vi "WF phase diversity_MATLAB_Correction_loop_1_Multi_3.vi"() -> ()   [LabVIEW 2018]
uses:
  Casao LabVIEW SDK 1.0.5/Casao/Casao/Casao.ctl
  <vilib>/Analysis/1siggen.llb/Ramp Pattern by Samples.vi
  <vilib>/Utility/file.llb/Read From Spreadsheet File (DBL).vi
  <vilib>/Analysis/1siggen.llb/Ramp Pattern by Delta.vi
  <vilib>/Analysis/NI_AALBase.lvlib
panel:
  in  "Tab Control":T1(tab)
  in  "Offset command file":path=path "D:/SystemAlignment/system_aberration_20200206.dat"
  in  "Initial haso file":path=path "D:/SystemAlignment/system_aberration_residual_20191015.has"
  in  "EMCCD trigger port":tag="Dev1/port0/line0"
  out "Casao Index":T2
  out "# of Phase":i32
  in  "Error in":errorcluster
  out "Error out":errorcluster
  in  "Initial Zer coeff":dbl[](array[numeric])=[0.2, 0.2]
  in  "Initial Zer index":dbl[](array[numeric])=[4.0, 5.0]
  out "Initial Zer coeff\nRandomly generated":dbl[](array[numeric])
  out "Initial Zer index (starting from 4)\nrandomly generated":dbl[](array[numeric])
  in  "aberration tolerance":dbl=0.1 format="%#_13g"
  in  "aberration threshold":dbl=0.25 format="%#_13g"
  in  "?":enum16{"input manually ", "randomly generated"}(ring)=enum."randomly generated"
  in  "max random order":i64=9
  in  "Data Acquisition Iteration #":i32=1
  in  "Zern index in 2":i32[](array[numeric])=[3, 4, 5, 6, 7, 8]
  in  "Zern coef in 2":sgl[](array[numeric])=[0.0, 0.0, 0.2, 0.0, 0.0, 0.0]
  in  "Zern index in 3":i32[](array[numeric])=[3, 4, 5, 6, 7, 8]
  in  "Zern coef in 3":sgl[](array[numeric])=[0.2, 0.0, 0.0, 0.0, 0.0, 0.0]
  in  "Zern index in 4":i32[](array[numeric])=[3, 4, 5, 6, 7, 8]
  in  "Zern coef in 4":sgl[](array[numeric])=[0.2, 0.0, 0.0, 0.0, 0.0, 0.0]
  in  "Zern index in 5":i32[](array[numeric])=[3, 4, 5, 6, 7, 8]
  in  "Zern coef in 5":sgl[](array[numeric])=[0.0, 0.0, 0.0, 0.0, 0.0, -0.2]
  in  "Andor Picture/notes save to path":path=path "D:/Data/20200214_PR_FixedCell/Cell1"
  in  "base name":string="beads_test"
  in  "Pics/phase":dbl=2.0
  in  "camera exposure time (s)":string="0.02"
  in  "# of Accumulations":string="1"
  in  "# of Phase":i32=5
  in  "Run Andor Codes?":bool
  in  "COMMAND matrix path":path=path "D:/SystemAlignment/IM_20200224.aomi"
  in  "ROI size":enum16{"full (1002*1002)", "512*512"}(ring)
  in  "take offset image?":bool=TRUE
  in  "Use GPU":bool=TRUE
  in  "Show Recon":bool=TRUE
  in  "Show Input":bool
  in  "Background Value":u32=290
  in  "Crop Size of image":u32=512
  in  "Gamma Value":dbl=1e-06
  in  "Iteration Number":u32=10
  in  "Zernike Order":u32=15
  in  "Number for average":u32=2
  in  "Number of Phase":u32=2
  in  "Run MATLAB or correction?":bool=TRUE
  in  "Keep Reconstructed Defocus component?":bool
  # "70"
  # "offset+aberr\nphase diversity\nground truth\noffset+aberr\ncorrected"
  # "Randomly Generate Initial Zernike, enter here:"
  # "Manually input, enter here:"
  # "Andor Camera Settings"
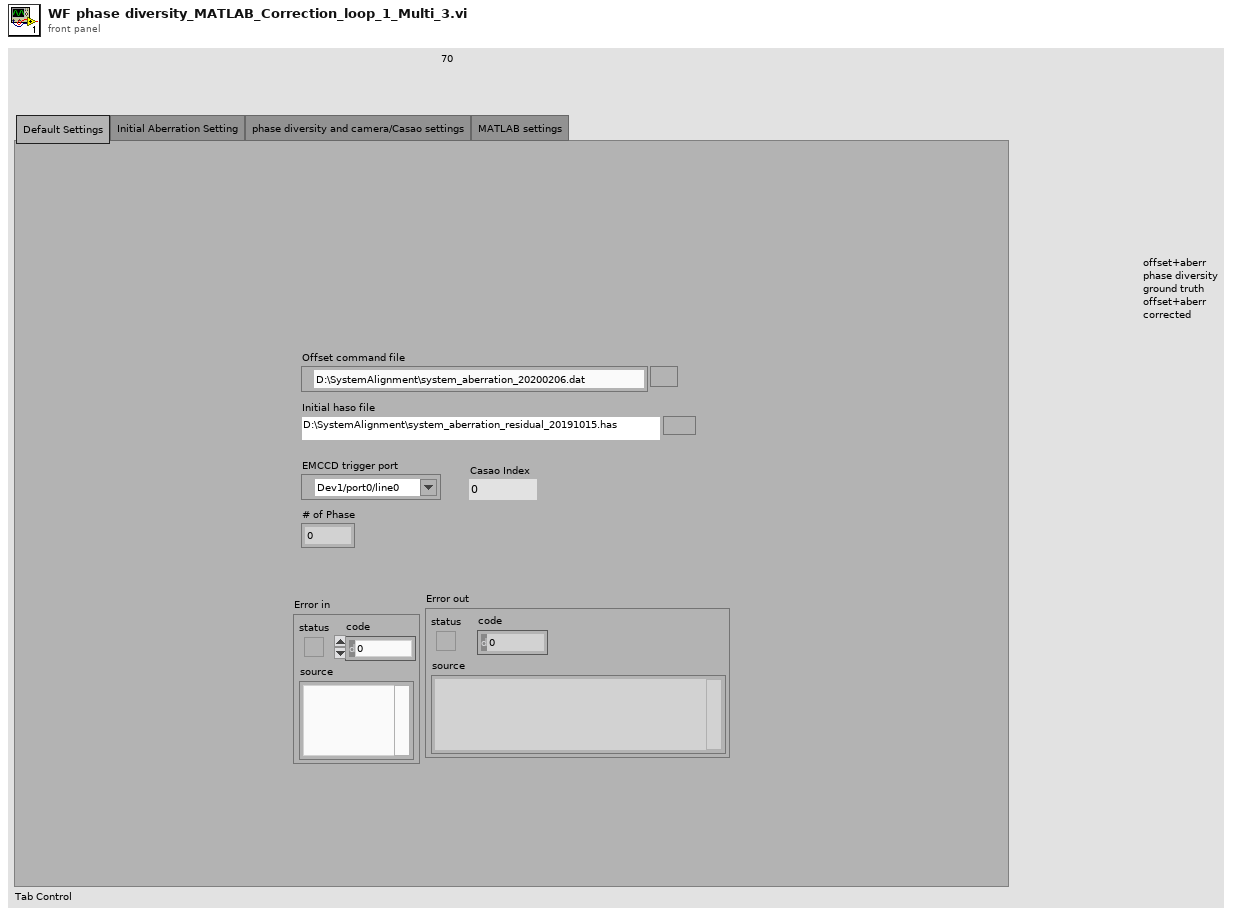
[diagram p1: front panel]
types:
  T1 = enum32{"Default Settings", "Initial Aberration Setting", "phase diversity and camera/Casao settings", "MATLAB settings"}
  T2 = typedef "Casao.ctl" = i32
  T3 = typedef "PhaseModul.ctl" = i32
  T4 = typedef "NI_Matrix.lvlib/RealMatrix.ctl" = dbl[][]
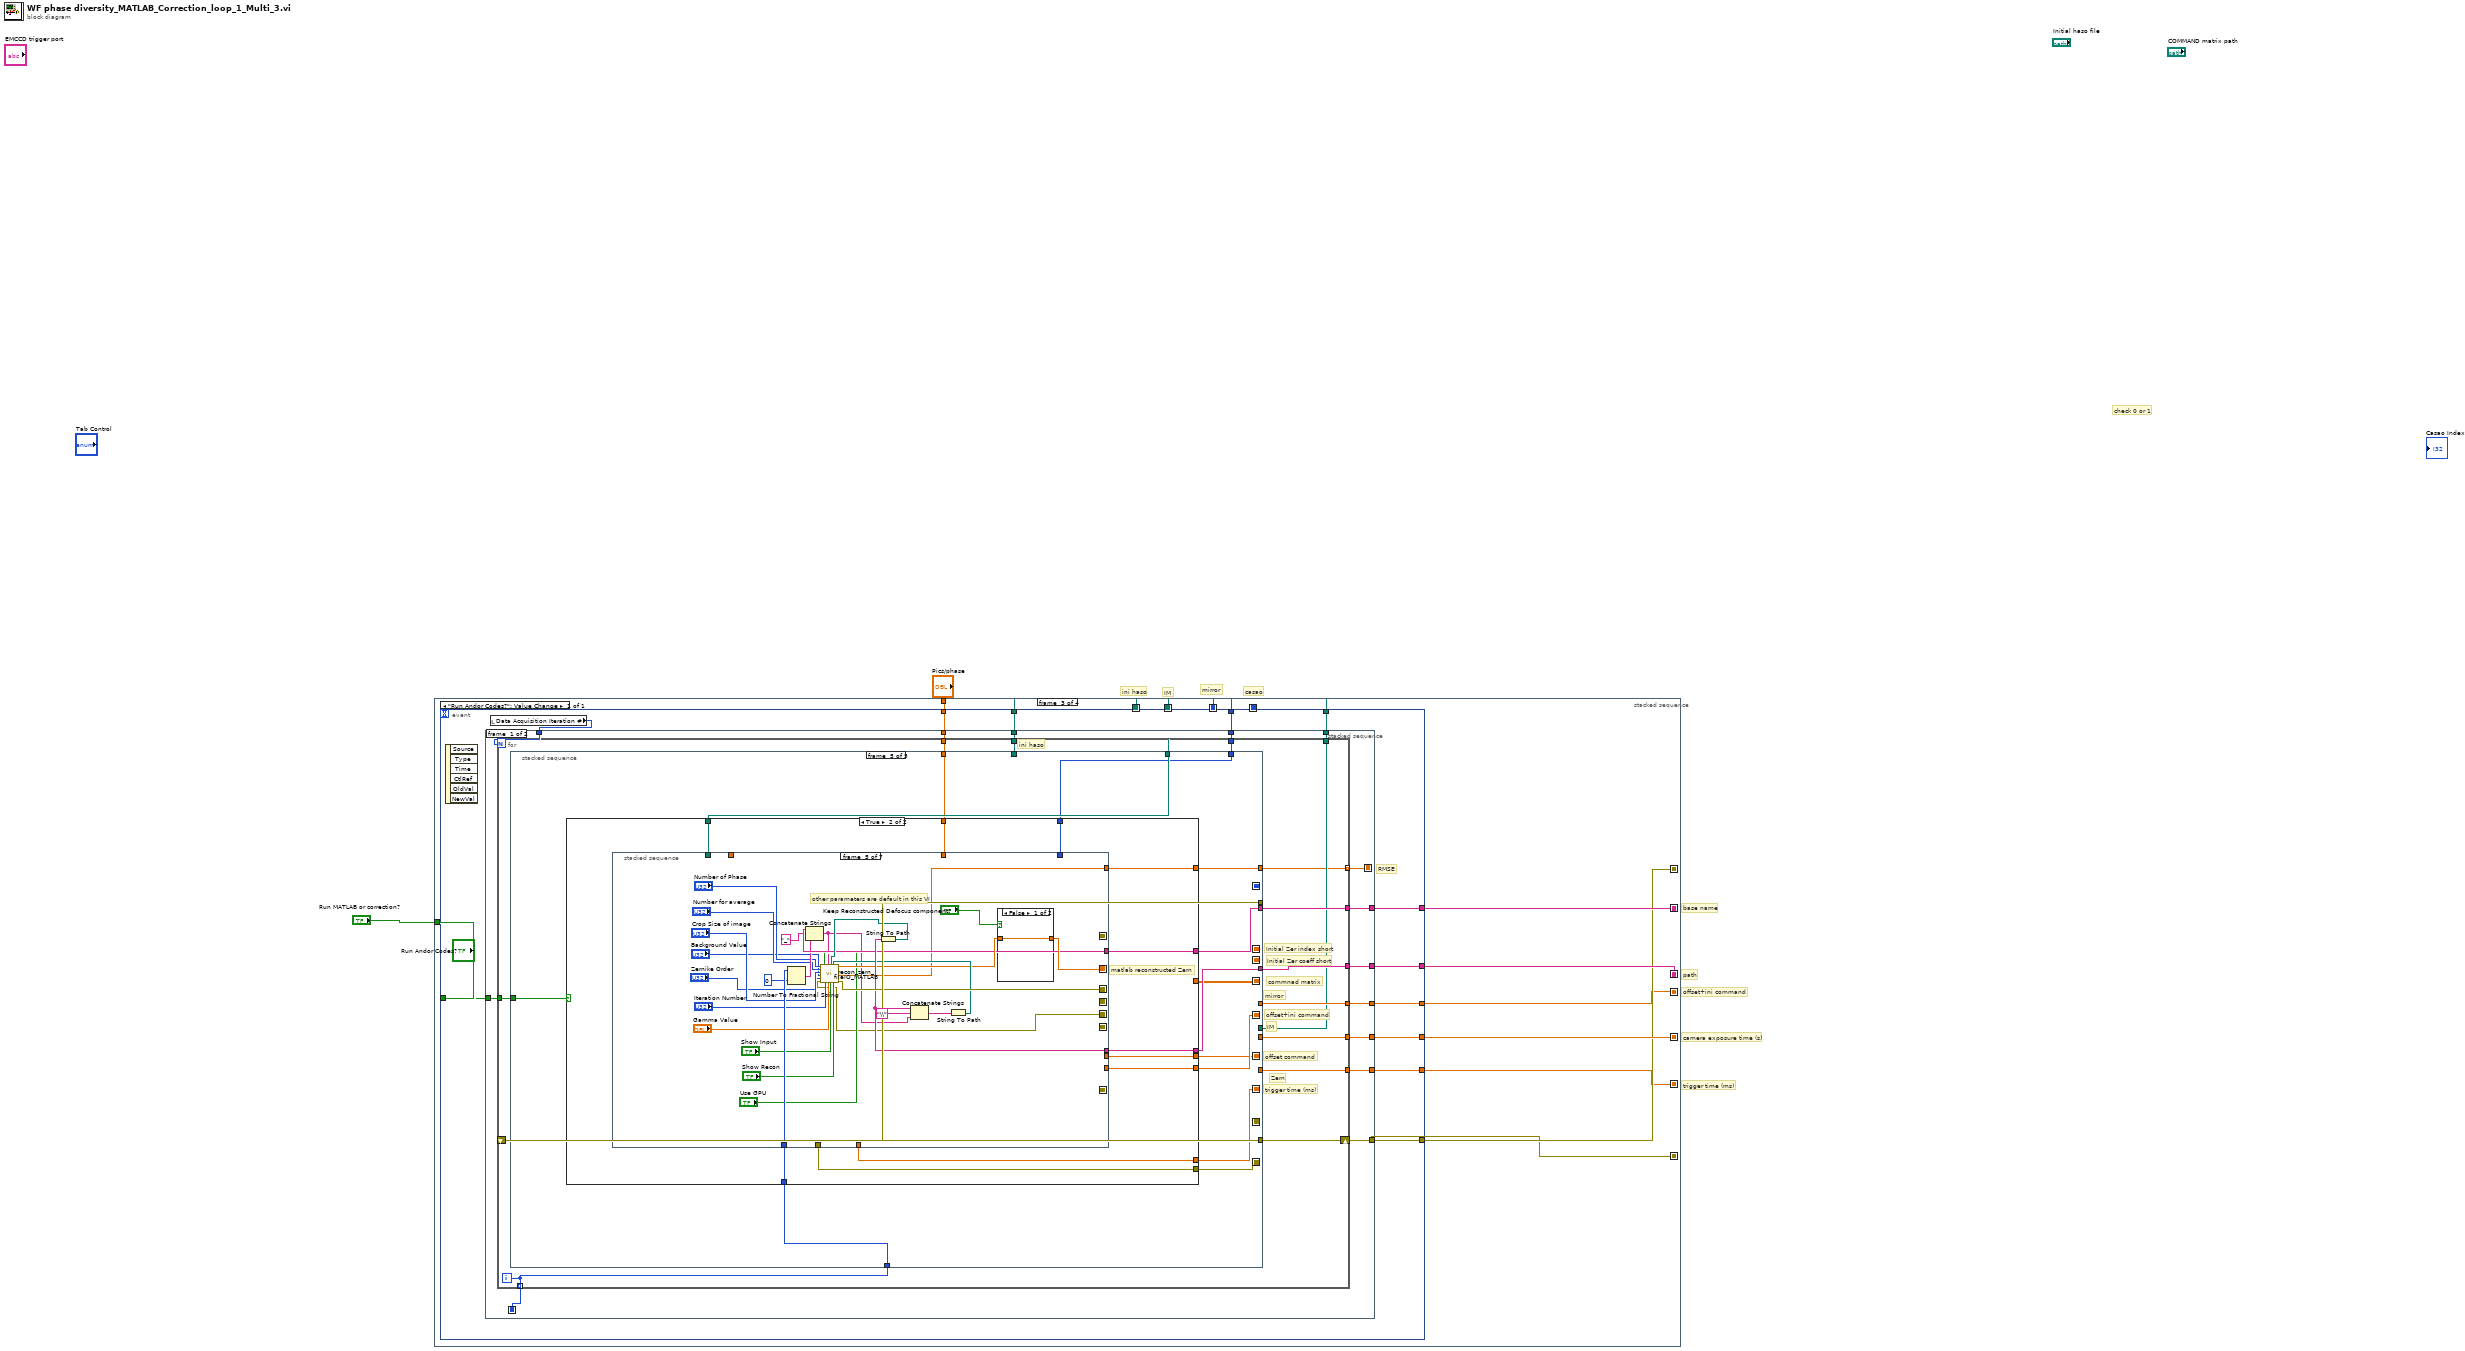
[diagram p0: block diagram]
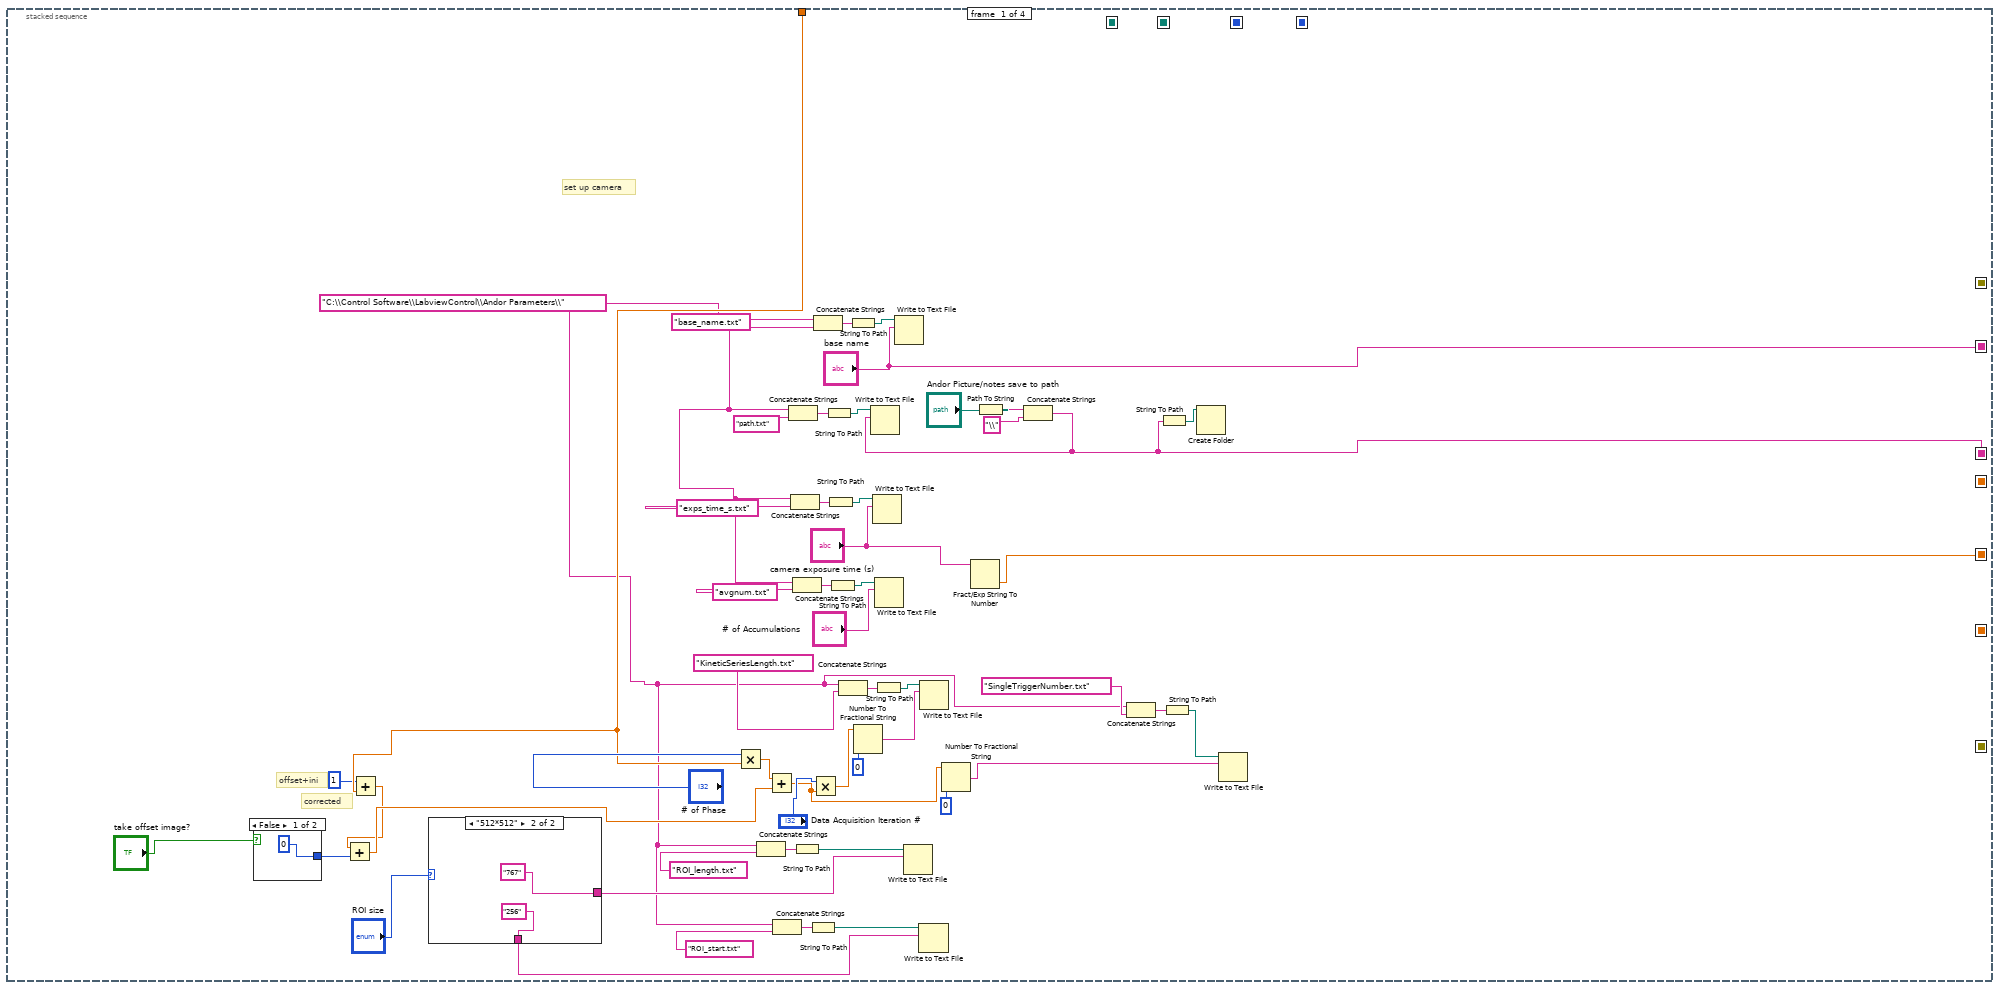
[diagram p2: hidden frame]
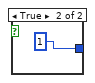
[diagram p3: hidden frame]
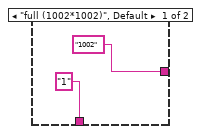
[diagram p4: hidden frame]
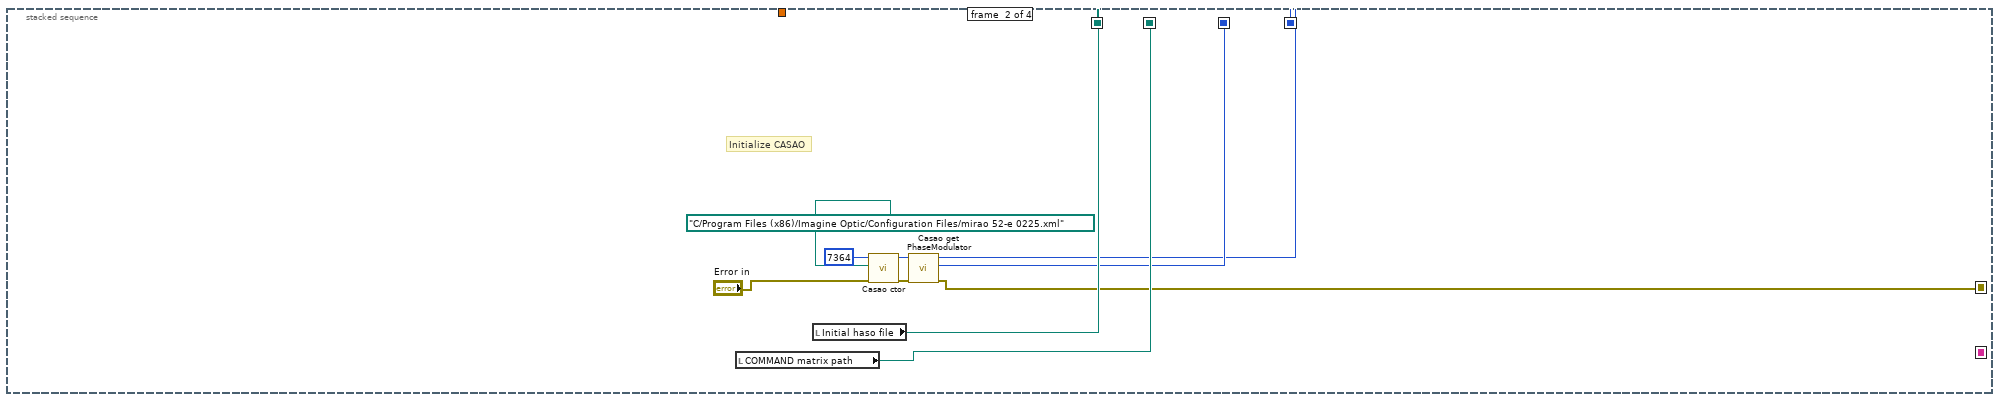
[diagram p5: hidden frame]
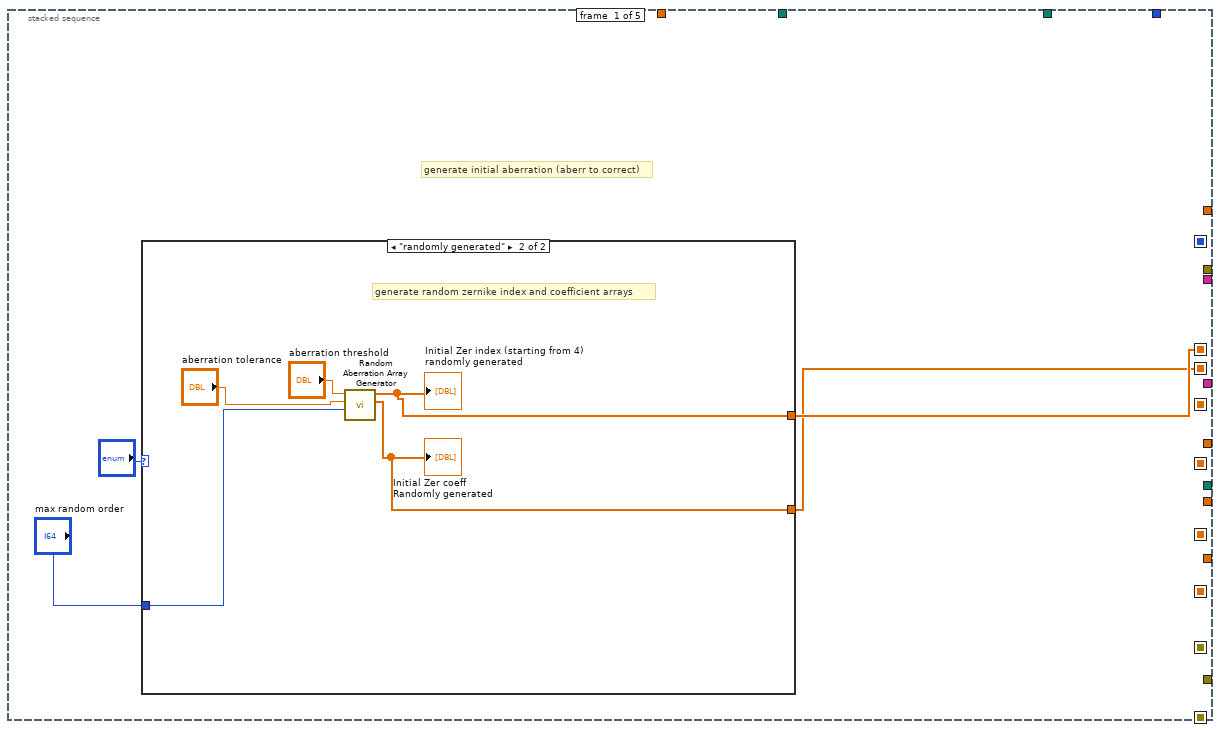
[diagram p6: hidden frame]
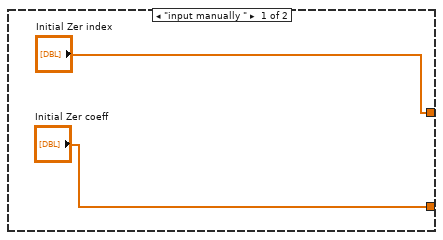
[diagram p7: hidden frame]
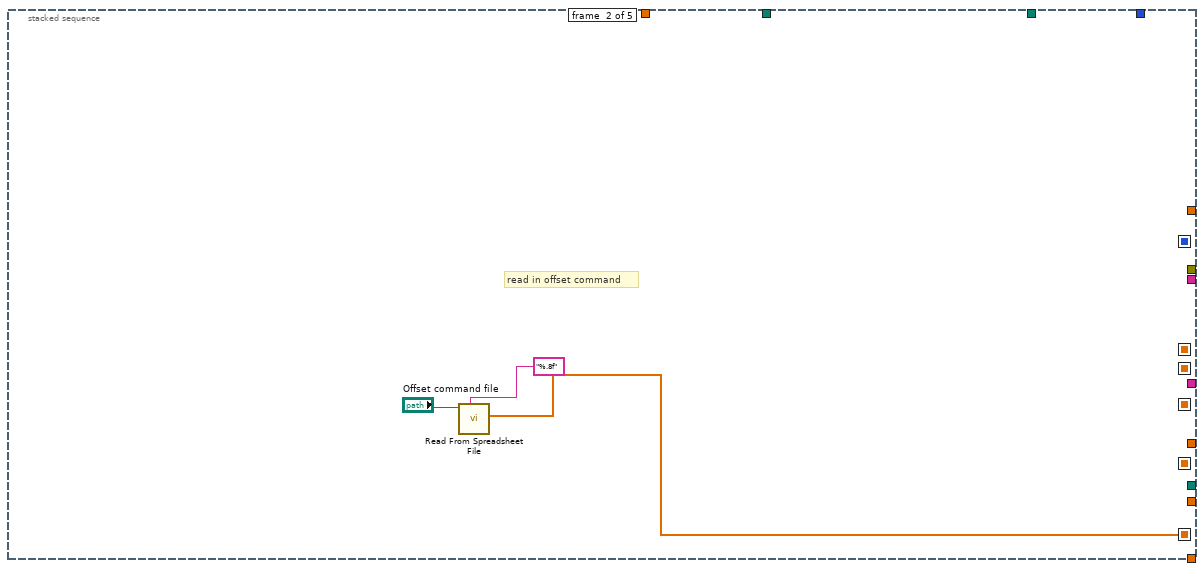
[diagram p8: hidden frame]
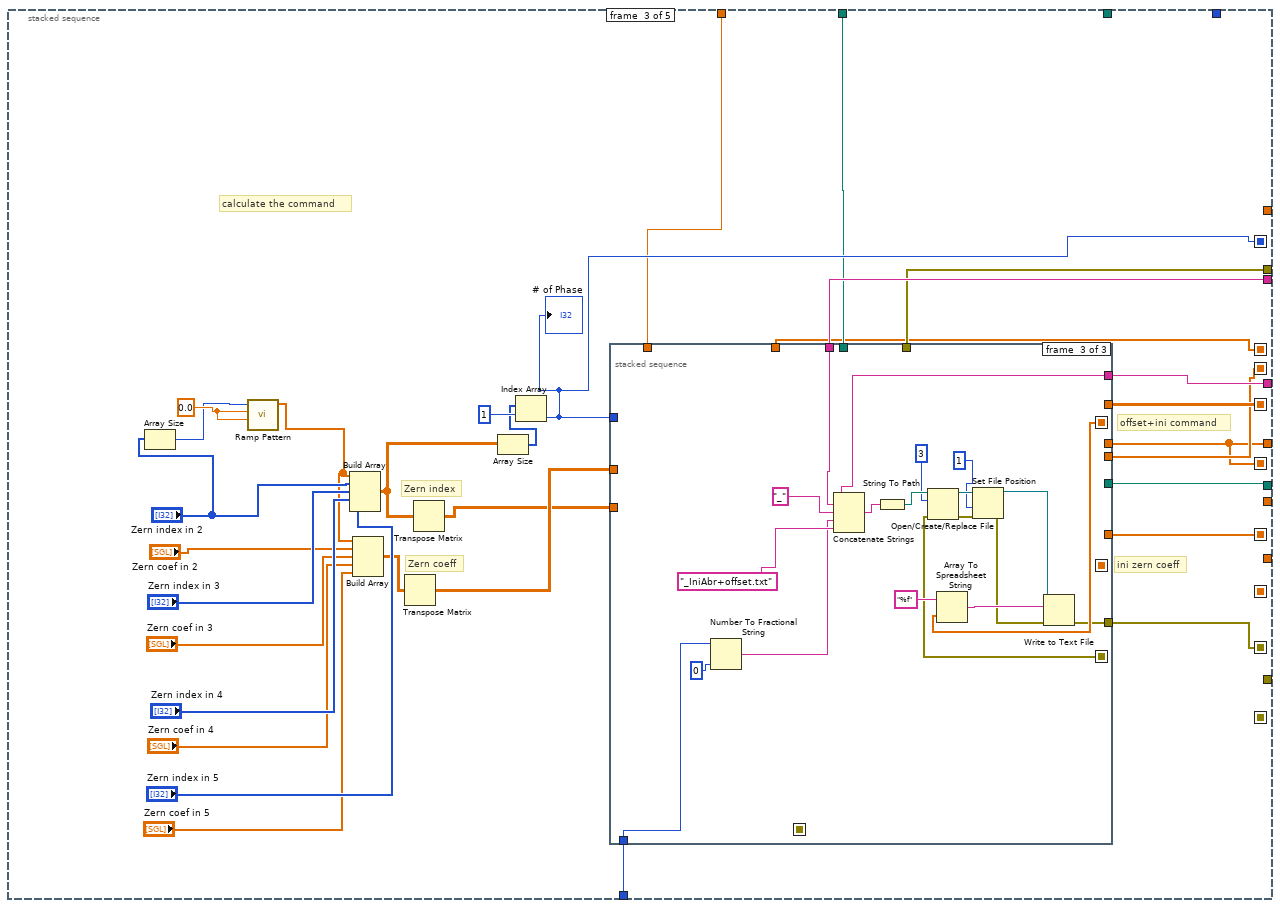
[diagram p9: hidden frame]
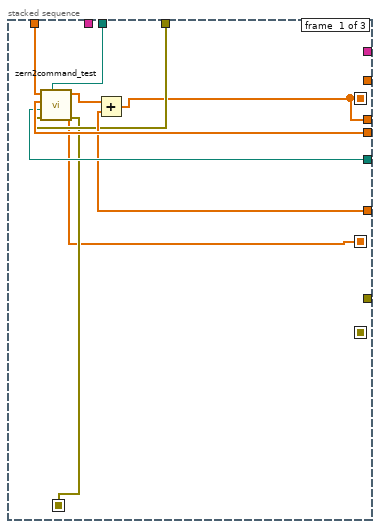
[diagram p10: hidden frame]
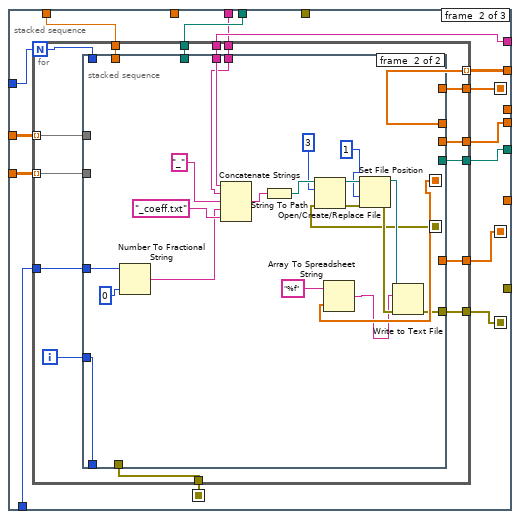
[diagram p11: hidden frame]
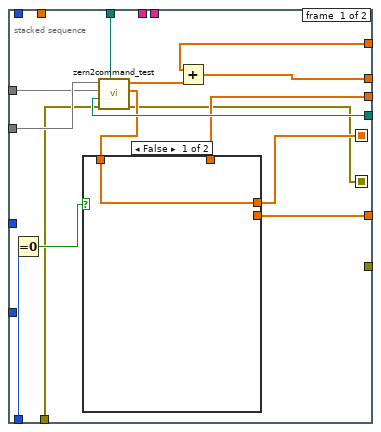
[diagram p12: hidden frame]
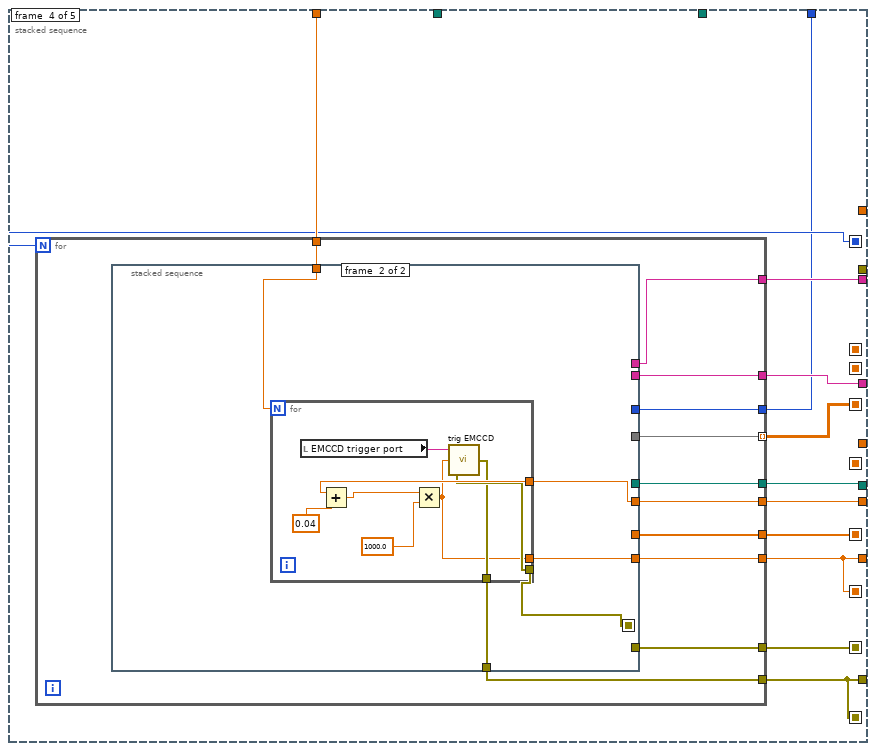
[diagram p14: hidden frame]
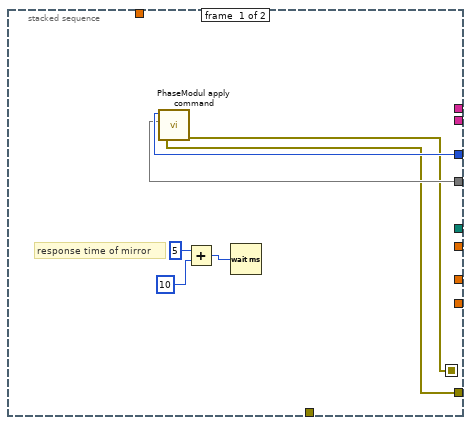
[diagram p15: hidden frame]
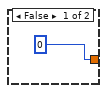
[diagram p16: hidden frame]
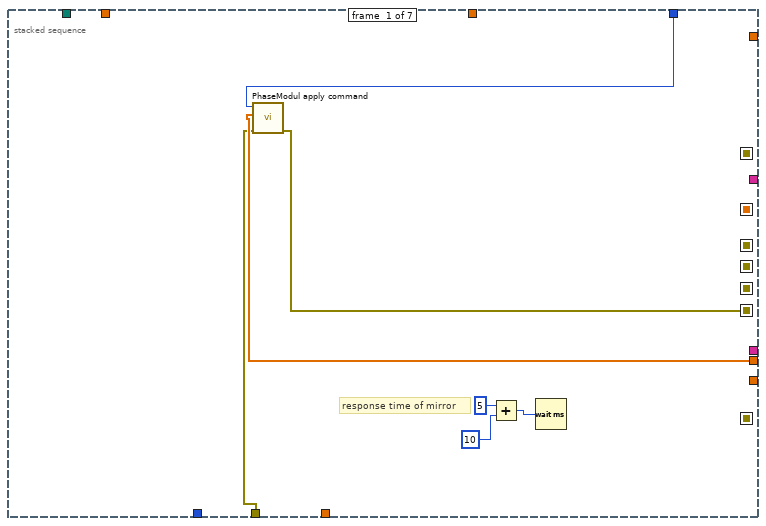
[diagram p17: hidden frame]
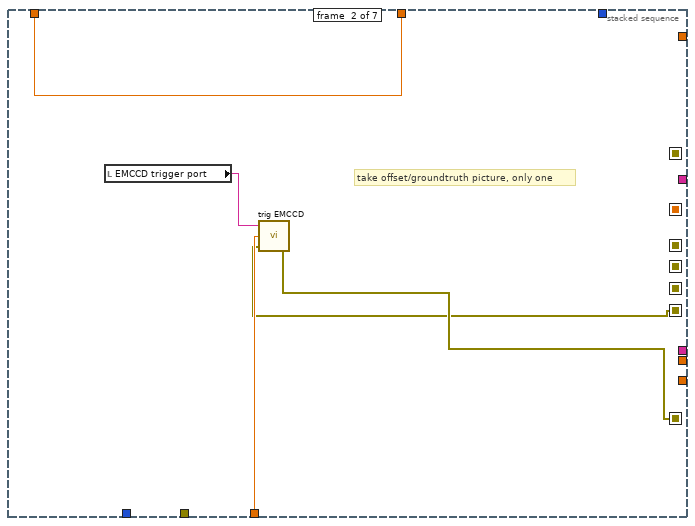
[diagram p18: hidden frame]
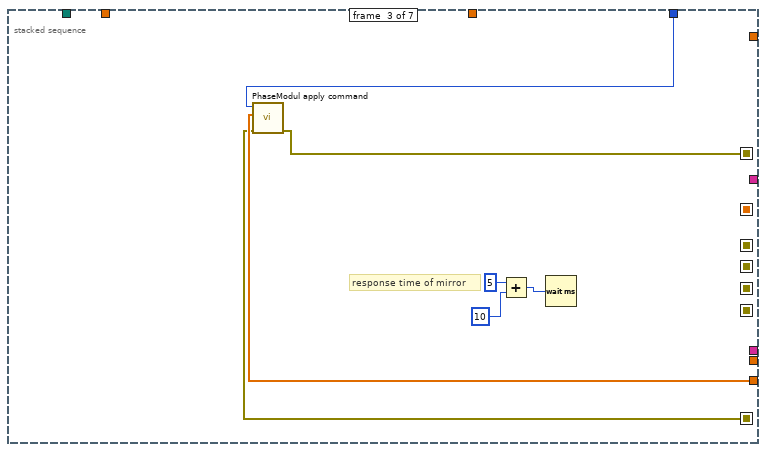
[diagram p19: hidden frame]
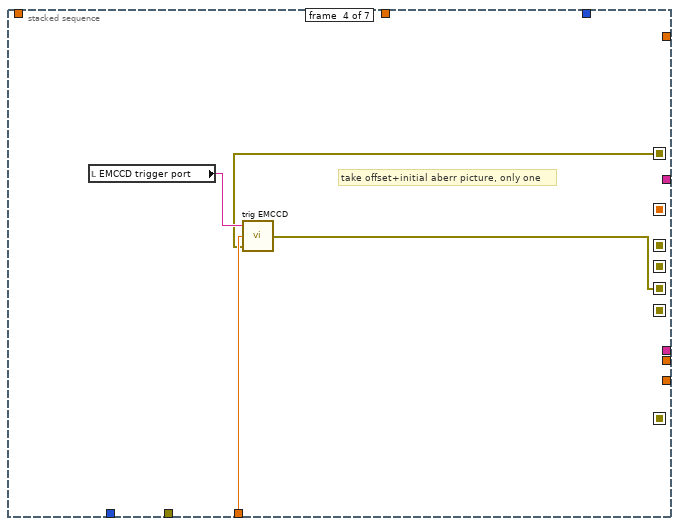
[diagram p20: hidden frame]
diagram:
  # "trigger time (ms)"
  # "offset+ini command"
  # "camera exposure time (s)"
  # "casao"
  # "mirror"
  # "IM"
  # "ini haso"
  # "path"
  # "base name"
  # "check 0 or 1"
  n1 = stacked-sequence {
    seq-local: [w14 _ _ _] -> [_ _ w81 _]
    seq-local: ["base name" _ _ _] -> [_ _ w80 _]
    seq-local: [_ w66 _ _] -> [_ _ w78 _]
    seq-local: [_ w65 _ _] -> [_ _ w72 _]
    seq-local: [_ w64 _ _] -> [_ _ w79 _]
    seq-local: [_ w63 _ _] -> [_ _ _ w421]
    seq-local: [w21 _ _ _] -> [_ _ w77 _]
    seq-local: [_ w61 _ _] -> [_ _ w76 _]
    seq-local: [_ _ w75 _] -> [_ _ _ _]
    seq-local: [_ _ w74 _] -> [_ _ _ _]
    seq-local: [_ _ w73 _] -> [_ _ _ _]
    tunnel: "Pics/phase" -> [w18 _ w82 _]
    tunnel: "Run MATLAB or correction?" -> [_ _ w71 _]
    frame #0 {
      w7 = "C:\\Control Software\\LabviewControl\\Andor Parameters\\"
      # "corrected"
      # "offset+ini"
      # "set up camera"
      n2 = case shown="False" "take offset image?" {
        tunnel: [0 1] -> w5
        frame False {
        }
        frame True {
        }
      }
      n3 = Add(x=1, y=w18) -> (x+y=w4:dbl)
      n4 = Add(x=w4, y=w5) -> (x+y=w19:dbl)
      n5 = case shown="\"512*512\"" "ROI size" {
        tunnel: ["1002" "767"] -> w27
        tunnel: ["1" "256"] -> w23
        frame "full (1002*1002)", Default {
        }
        frame "512*512" {
        }
      }
      n6 = Multiply(x="# of Phase", y=w18) -> (x*y=w20:dbl)
      n7 = Concatenate Strings(w7, "ROI_length.txt") -> (w31:string)
      n8 = Add(x=w20, y=w19) -> (x+y=w12:dbl)
      n9 = Concatenate Strings(w7, "ROI_start.txt") -> (w26:string)
      n10 = Concatenate Strings(w7, "path.txt") -> (w51:string)
      n11 = Concatenate Strings(w7, "exps_time_s.txt") -> (w48:string)
      n12 = Concatenate Strings(w7, "avgnum.txt") -> (w45:string)
      n13 = String To Path(string=w31) -> (path=w30:path)
      n14 = String To Path(string=w26) -> (path=w25:path)
      n15 = Multiply(x="Data Acquisition Iteration #", y=w12) -> (x*y=w16:dbl)
      n16 = Concatenate Strings(w7, "base_name.txt") -> (w53:string)
      n17 = String To Path(string=w51) -> (path=w50:path)
      n18 = String To Path(string=w48) -> (path=w47:path)
      n19 = String To Path(string=w45) -> (path=w44:path)
      n20 = Concatenate Strings(w7, "KineticSeriesLength.txt") -> (w41:string)
      n21 = String To Path(string=w53) -> (path=w52:path)
      n22 = Number To Fractional String(number=w16, precision (6)=0) -> (F-format string=w38:string)  [unwired: 2 in]
      n23 = Write to Text File(file (use dialog)=w47, text="camera exposure time (s)") -> ()  [unwired: 2 in, 3 out]
      n24 = Write to Text File(file (use dialog)=w44, text="# of Accumulations") -> ()  [unwired: 2 in, 3 out]
      n25 = String To Path(string=w41) -> (path=w40:path)
      n26 = Write to Text File(file (use dialog)=w52, text="base name") -> ()  [unwired: 2 in, 3 out]
      n27 = Write to Text File(file (use dialog)=w30, text=w27) -> ()  [unwired: 2 in, 3 out]
      n28 = Write to Text File(file (use dialog)=w25, text=w23) -> ()  [unwired: 2 in, 3 out]
      n29 = Write to Text File(file (use dialog)=w40, text=w38) -> ()  [unwired: 2 in, 3 out]
      n30 = Number To Fractional String(number=w12, precision (6)=0) -> (F-format string=w11:string)  [unwired: 2 in]
      n31 = Fract/Exp String To Number(string="camera exposure time (s)") -> (number=w21:dbl)  [unwired: 3 in, 1 out]
      n32 = Path To String(path="Andor Picture/notes save to path") -> (string=w33:string)
      n33 = Concatenate Strings(w33, "\\") -> (w14:string)
      n34 = Write to Text File(file (use dialog)=w50, text=w14) -> ()  [unwired: 2 in, 3 out]
      n35 = Concatenate Strings(w7, "SingleTriggerNumber.txt") -> (w10:string)
      n36 = String To Path(string=w14) -> (path=w15:path)
      n37 = String To Path(string=w10) -> (path=w9:path)
      n38 = Create Folder(path (use dialog)=w15) -> ()  [unwired: 2 in, 3 out]
      n39 = Write to Text File(file (use dialog)=w9, text=w11) -> ()  [unwired: 2 in, 3 out]
    }
    frame #1 {
      # "Initialize CASAO"
      n40 = local read "COMMAND matrix path"() -> (w65:path)
      n41 = local read "Initial haso file"() -> (w66:path)
      n42 = call "Casao ctor.vi"("error in (no error)"="Error in", "Mirror config file path"=path "C:/Program Files (x86)/Imagine Optic/Configuration Files/mirao 52-e 0225.xml", "Haso serial number"=u32 7364) -> ("error out"=w70:errorcluster, "Casao"=w69:T2)  [unwired: 5 in]
      n43 = call "Casao get PhaseModulator.vi"("error in (no error)"=w70, "Casao"=w69) -> ("error out"=w61:errorcluster, "Mirrror"=w64:T3, "Casao (dup)"=w63:T2)  [unwired: 3 in]
    }
    frame #2 {
      n44 = event shown="[0] \"Run Andor Codes?\": Value Change" {
        selector: _ -> [_]
        dyn-events: _ -> [_]
        timeout: _ -> [_]
        tunnel: w82 -> [w95]
        tunnel: w81 -> [w94]
        tunnel: w80 -> [w93]
        tunnel: w79 -> [w92]
        tunnel: w78 -> [w91]
        tunnel: w77 -> [w90]
        tunnel: w76 -> [w89]
        tunnel: [w88] -> w75
        tunnel: [w87] -> w74
        tunnel: [w86] -> w73
        tunnel: w72 -> [w85]
        tunnel: w71 -> [w84]
        event "Run Andor Codes?": Value Change {
          # "RMSE"
          n45 = event-data() -> ()  [unwired: 1 in, 6 out]
          n46 = local read "Data Acquisition Iteration #"() -> (w83:i32)
          n47 = stacked-sequence {
            seq-local: [w97 _] -> [_ w416]
            seq-local: [w96 _] -> [_ _]
            tunnel: w95 -> [w110 _]
            tunnel: w94 -> [w109 w415]
            tunnel: w93 -> [w108 w414]
            tunnel: w92 -> [w107 _]
            tunnel: w91 -> [w106 _]
            tunnel: w90 -> [w105 _]
            tunnel: w89 -> [w104 _]
            tunnel: [w103 _] -> w88
            tunnel: [w102 _] -> w87
            tunnel: [w101 _] -> w86
            tunnel: w85 -> [w100 _]
            tunnel: w84 -> [w99 _]
            tunnel: w83 -> [w98 _]
            frame #0 {
              n48 = for {
                N: w98 -> [_]
                tunnel: w110 -> [w124]
                tunnel: w109 -> [w123]
                tunnel: w108 -> [w122]
                tunnel: w107 -> [w121]
                tunnel: w106 -> [w120]
                tunnel: w105 -> [w119]
                tunnel: [w117] -> w103
                tunnel: [w116] -> w102
                tunnel: w100 -> [w114]
                tunnel: w99 -> [w113]
                shift-right: [w115] -> w101
                shift-left: w104 -> [w118]
                tunnel: [w112] -> w97 mode=indexing
                tunnel: [w111] -> w96 mode=indexing
                i -> [w111]
                # "trigger time (ms)"
                # "offset+ini command"
                # "Initial Zer coeff short"
                # "Initial Zer index short"
                # "mirror"
                # "Zern"
                # "commnad matrix"
                # "ini haso"
                # "IM"
                # "offset command"
                n49 = stacked-sequence {
                  seq-local: [_ w136 _ _ _] -> [_ _ w156 w276 w311]
                  seq-local: [_ _ w154 _ _] -> [_ _ _ w275 w313]
                  seq-local: [_ _ w152 _ _] -> [_ _ _ w274 _]
                  seq-local: [_ _ w145 _ _] -> [_ _ _ w270 _]
                  seq-local: [w127 _ _ _ _] -> [_ _ w142 _ _]
                  seq-local: [w126 _ _ _ _] -> [_ _ w141 _ _]
                  seq-local: [_ _ w140 _ _] -> [_ _ _ _ w320]
                  seq-local: [_ _ _ w269 _] -> [_ _ _ _ w317]
                  seq-local: [_ _ _ w268 _] -> [_ _ _ _ w316]
                  tunnel: w124 -> [_ _ w149 w279 w318]
                  tunnel: w123 -> [_ _ w150 w278 w322]
                  tunnel: w122 -> [_ _ w151 w277 w323]
                  tunnel: w120 -> [_ _ w148 _ _]
                  tunnel: w114 -> [_ _ w147 w273 _]
                  tunnel: w121 -> [_ _ _ w272 w319]
                  tunnel: w119 -> [_ _ _ w271 _]
                  tunnel: w118 -> [_ _ w146 _ _]
                  tunnel: [_ _ _ w268 _] -> w115
                  tunnel: [_ _ w140 _ _] -> w117
                  tunnel: [_ _ _ w269 _] -> w116
                  tunnel: w114 -> [_ _ _ _ w321]
                  tunnel: w113 -> [_ _ _ _ w315]
                  tunnel: w111 -> [_ _ w139 _ w314]
                  tunnel: [_ _ _ _ w312] -> w112
                  frame #0 {
                    # "generate initial aberration (aberr to correct)"
                    n50 = case shown="\"randomly generated\"" "?" {
                      tunnel: ["Initial Zer index" w133] -> w127
                      tunnel: ["Initial Zer coeff" w132] -> w126
                      tunnel: "max random order" -> [_ w131]
                      frame "input manually " {
                      }
                      frame "randomly generated" {
                        # "generate random zernike index and coefficient arrays"
                        n51 = call "Random Aberration Array Generator.vi"("max random order"=w131, "aberration tolerance"="aberration tolerance", "aberration threshold"="aberration threshold") -> ("Zer coeff"=w132:dbl[], "Zer index (starting from 3)"=w133:dbl[])  [unwired: 7 in]
                        "Initial Zer index (starting from 4)\nrandomly generated" <- w133
                        "Initial Zer coeff\nRandomly generated" <- w132
                      }
                    }
                  }
                  frame #1 {
                    # "read in offset command"
                    n52 = call-poly <vilib>:"Read From Spreadsheet File.vi"("format (%.3f)"="%.8f", "file path (dialog if empty)"="Offset command file") -> ("first row"=w136:dbl[])  [unwired: 5 in, 4 out]
                  }
                  frame #2 {
                    w161 = 0.0
                    # "ini zern coeff"
                    # "offset+ini command"
                    # "Zern coeff"
                    # "Zern index"
                    # "calculate the command"
                    n53 = Array Size(array="Zern index in 2") -> (size(s)=w159:i32)
                    n54 = call-poly <vilib>:"Ramp Pattern.vi"("start"=w161, "end"=w161, "samples"=w159) -> ("Ramp Pattern"=w158:dbl[])  [unwired: 7 in, 1 out]
                    n55 = Build Array(w158, "Zern index in 2", "Zern index in 3", "Zern index in 4", "Zern index in 5") -> (w143:T4)
                    n56 = Build Array(w158, "Zern coef in 2", "Zern coef in 3", "Zern coef in 4", "Zern coef in 5") -> (w162:T4)
                    n57 = Transpose Matrix(1:w162) -> (0:w155:T4)
                    n58 = Transpose Matrix(1:w143) -> (0:w153:T4)
                    n59 = Array Size(array=w143) -> (size(s)=w144:i32[])
                    n60 = Index Array(array=w144, index=1) -> (element=w152:i32)
                    "# of Phase" <- w152
                    n61 = stacked-sequence {
                      seq-local: [w171 _ _] -> [_ w189 w255]
                      seq-local: [w172 _ _] -> [_ w183 _]
                      seq-local: [_ w182 _] -> [_ _ w252]
                      seq-local: [w170 _ _] -> [_ w181 _]
                      tunnel: w152 -> [_ w194 _]
                      tunnel: w142 -> [w179 _ _]
                      tunnel: w141 -> [w178 w184 _]
                      tunnel: w147 -> [w177 w191 _]
                      tunnel: w156 -> [w175 _ _]
                      tunnel: w153 -> [_ w193 _]
                      tunnel: w155 -> [_ w192 _]
                      tunnel: w148 -> [w174 w190 _]
                      tunnel: [_ w188 _] -> w154
                      tunnel: w151 -> [_ w186 w253]
                      tunnel: w150 -> [_ w187 w254]
                      tunnel: w149 -> [_ w185 _]
                      tunnel: w146 -> [w173 _ _]
                      tunnel: [_ _ w251] -> w145
                      tunnel: [w171 _ _] -> w140
                      tunnel: w139 -> [_ w180 w249]
                      frame #0 {
                        n62 = call "zern2command_test.vi"("Initial haso file"=w174, "error in (no error)"=w173, "interaction matrix file"=w177, "Zern coef in"=w178, "Zern index in"=w179) -> ("error out"=w172:errorcluster, "Zern coef out"=w170:sgl[], "Offset positions"=w176:sgl[])  [unwired: 4 in]
                        n63 = Add(x=w176, y=w175) -> (x+y=w171:dbl[])
                      }
                      frame #1 {
                        n64 = for {
                          N: w194 -> [w197]
                          tunnel: w193 -> [w210] mode=indexing
                          tunnel: w192 -> [w209] mode=indexing
                          tunnel: w191 -> [w208]
                          tunnel: w190 -> [w207]
                          tunnel: w189 -> [w206]
                          tunnel: [w205] -> w188 mode=indexing
                          tunnel: w187 -> [w204]
                          tunnel: w186 -> [w203]
                          tunnel: w185 -> [w202]
                          tunnel: w184 -> [w201]
                          tunnel: w183 -> [w200]
                          tunnel: [w199] -> w182
                          tunnel: w181 -> [w196]
                          tunnel: w180 -> [w195]
                          i -> [w198]
                          n65 = stacked-sequence {
                            seq-local: [w216 _] -> [_ w235]
                            seq-local: [w212 _] -> [_ w234]
                            tunnel: w210 -> [w225 _]
                            tunnel: w209 -> [w224 _]
                            tunnel: w208 -> [w223 _]
                            tunnel: w207 -> [w222 _]
                            tunnel: w206 -> [w220 _]
                            tunnel: [w219 _] -> w205
                            tunnel: w204 -> [_ w237]
                            tunnel: w203 -> [_ w236]
                            tunnel: w202 -> [_ _]
                            tunnel: w198 -> [w218 _]
                            tunnel: w201 -> [w214 _]
                            tunnel: w200 -> [w213 _]
                            tunnel: [_ w233] -> w199
                            tunnel: w198 -> [_ _]
                            tunnel: w197 -> [_ _]
                            tunnel: w196 -> [w211 _]
                            tunnel: w195 -> [_ w230]
                            frame #0 {
                              n66 = Equal To 0?(x=w218) -> (x = 0?=w217:bool)
                              n67 = call "zern2command_test.vi"("Initial haso file"=w222, "error in (no error)"=w213, "interaction matrix file"=w223, "Zern coef in"=w224, "Zern index in"=w225) -> ("error out"=w212:errorcluster, "Zern coef out"=w215:sgl[], "Offset positions"=w221:sgl[])  [unwired: 4 in]
                              n68 = case shown="False" w217 {
                                tunnel: [w226 w227] -> w216
                                tunnel: w215 -> [w226 _]
                                tunnel: w214 -> [_ _]
                                tunnel: w211 -> [_ w227]
                                frame False {
                                }
                                frame True {
                                }
                              }
                              n69 = Add(x=w220, y=w221) -> (x+y=w219:dbl[])
                            }
                            frame #1 {
                              n70 = Number To Fractional String(number=w230, precision (6)=0) -> (F-format string=w229:string)  [unwired: 2 in]
                              n71 = Concatenate Strings(w237, w236, "_", w229, "_coeff.txt") -> (w245:string)
                              n72 = String To Path(string=w245) -> (path=w244:path)
                              n73 = Open/Create/Replace File(file path (use dialog)=w244, error in=w234, operation (0:open)=3) -> (refnum out=w241:refnum<file>, error out=w242:errorcluster)  [unwired: 3 in, 1 out]
                              n74 = Array To Spreadsheet String(array=w235, 3:"%f") -> (spreadsheet string=w232:string)  [unwired: 1 in]
                              n75 = Set File Position(refnum=w241, from (0:start)=1, error in=w242) -> (refnum out=w239:refnum<file>, error out=w238:errorcluster)  [unwired: 1 in]
                              n76 = Write to Text File(file (use dialog)=w239, text=w232, error in=w238) -> (error out=w233:errorcluster)  [unwired: 1 in, 2 out]
                            }
                          }
                        }
                      }
                      frame #2 {
                        n77 = Number To Fractional String(number=w249, precision (6)=0) -> (F-format string=w248:string)  [unwired: 2 in]
                        n78 = Concatenate Strings(w254, w253, "_", w248, "_IniAbr+offset.txt") -> (w264:string)
                        n79 = String To Path(string=w264) -> (path=w262:path)
                        n80 = Open/Create/Replace File(file path (use dialog)=w262, error in=w252, operation (0:open)=3) -> (refnum out=w259:refnum<file>, error out=w260:errorcluster)  [unwired: 3 in, 1 out]
                        n81 = Array To Spreadsheet String(array=w255, 3:"%f") -> (spreadsheet string=w266:string)  [unwired: 1 in]
                        n82 = Set File Position(refnum=w259, from (0:start)=1, error in=w260) -> (refnum out=w257:refnum<file>, error out=w256:errorcluster)  [unwired: 1 in]
                        n83 = Write to Text File(file (use dialog)=w257, text=w266, error in=w256) -> (error out=w251:errorcluster)  [unwired: 1 in, 2 out]
                      }
                    }
                  }
                  frame #3 {
                    n84 = for {
                      N: w274 -> [_]
                      tunnel: w279 -> [w290]
                      tunnel: w278 -> [w289]
                      tunnel: w277 -> [w288]
                      tunnel: w273 -> [w287]
                      tunnel: w276 -> [w286]
                      tunnel: w272 -> [w285]
                      tunnel: w275 -> [w284] mode=indexing
                      tunnel: w271 -> [w283]
                      tunnel: w270 -> [w282]
                      tunnel: [w281] -> w268
                      tunnel: [w280] -> w269
                      n85 = stacked-sequence {
                        seq-local: [w291 _] -> [_ w300]
                        tunnel: w290 -> [_ w302]
                        tunnel: w289 -> [_ _]
                        tunnel: w288 -> [_ _]
                        tunnel: w287 -> [_ _]
                        tunnel: w286 -> [_ _]
                        tunnel: w285 -> [w297 _]
                        tunnel: w284 -> [w296 _]
                        tunnel: w283 -> [_ w301]
                        tunnel: w282 -> [w292 _]
                        tunnel: [_ w299] -> w281
                        tunnel: [_ w298] -> w280
                        frame #0 {
                          # "response time of mirror"
                          n86 = call "PhaseModul apply command.vi"("error in (no error)"=w292, "Commands in"=w296, "Mirror"=w297) -> ("error out"=w291:errorcluster)  [unwired: 2 in, 2 out]
                          n87 = Add(x=5, y=10) -> (x+y=w293:i32)
                          n88 = Wait (ms)(milliseconds to wait=w293) -> ()  [unwired: 1 out]
                        }
                        frame #1 {
                          n89 = for {
                            N: w302 -> [_]
                            tunnel: w301 -> [w307]
                            tunnel: w300 -> [w305]
                            tunnel: [w304] -> w299
                            tunnel: [w303] -> w298
                            n90 = local read "EMCCD trigger port"() -> (w310:tag)
                            n91 = Add(x=w307, y=0.04) -> (x+y=w306:dbl)
                            n92 = Multiply(x=w306, y=1000.0) -> (x*y=w303:dbl)
                            n93 = call "trig EMCCD.vi"("error in (no error)"=w305, "exp time (ms)"=w303, "lines"=w310) -> ("error out"=w304:errorcluster)
                          }
                        }
                      }
                    }
                  }
                  frame #4 {
                    n94 = case shown="True" w315 {
                      tunnel: w322 -> [_ w335]
                      tunnel: w323 -> [_ w334]
                      tunnel: w321 -> [_ w333]
                      tunnel: w320 -> [_ w332]
                      tunnel: w319 -> [_ w331]
                      tunnel: w317 -> [_ w330]
                      tunnel: w318 -> [_ w329]
                      tunnel: w316 -> [_ w328]
                      tunnel: w314 -> [_ w327]
                      tunnel: w313 -> [_ _]
                      tunnel: [0 w326] -> w312
                      tunnel: w311 -> [_ w325]
                      frame False {
                      }
                      frame True {
                        # "matlab reconstructed Zern"
                        n95 = stacked-sequence {
                          seq-local: [_ _ _ _ w377 _ _] -> [_ _ _ _ _ w402 _]
                          seq-local: [_ _ _ _ w384 _ _] -> [_ _ _ _ _ w396 _]
                          seq-local: [_ _ w348 _ _ _ _] -> [_ _ _ w356 _ _ _]
                          seq-local: [w341 _ _ _ _ _ _] -> [_ w343 _ _ _ _ _]
                          seq-local: [_ w345 _ _ _ _ _] -> [_ _ w352 _ _ _ _]
                          seq-local: [_ _ _ w355 _ _ _] -> [_ _ _ _ w359 _ _]
                          seq-local: [_ _ _ _ _ w391 _] -> [_ _ _ _ _ _ w406]
                          tunnel: w335 -> [_ _ _ _ w383 _ _]
                          tunnel: w334 -> [_ _ _ _ w376 _ _]
                          tunnel: w333 -> [_ _ _ _ _ w401 _]
                          tunnel: w332 -> [_ _ w353 _ _ w400 _]
                          tunnel: w331 -> [w342 _ w354 _ _ w398 _]
                          tunnel: w330 -> [_ w347 _ w358 _ _ w409]
                          tunnel: w328 -> [w336 _ _ _ _ _ _]
                          tunnel: [_ w346 _ _ _ _ _] -> _
                          tunnel: w329 -> [_ w346 _ _ _ _ w408]
                          tunnel: w327 -> [_ _ _ _ w374 _ _]
                          tunnel: [_ _ _ _ w360 _ _] -> w326
                          tunnel: w325 -> [w340 _ _ _ _ _ _]
                          frame #0 {
                            # "response time of mirror"
                            n96 = call "PhaseModul apply command.vi"("error in (no error)"=w336, "Commands in"=w340, "Mirror"=w342) -> ("error out"=w341:errorcluster)  [unwired: 2 in, 2 out]
                            n97 = Add(x=5, y=10) -> (x+y=w337:i32)
                            n98 = Wait (ms)(milliseconds to wait=w337) -> ()  [unwired: 1 out]
                          }
                          frame #1 {
                            # "take offset/groundtruth picture, only one"
                            n99 = local read "EMCCD trigger port"() -> (w344:tag)
                            n100 = call "trig EMCCD.vi"("error in (no error)"=w343, "exp time (ms)"=w347, "lines"=w344) -> ("error out"=w345:errorcluster)
                          }
                          frame #2 {
                            # "response time of mirror"
                            n101 = call "PhaseModul apply command.vi"("error in (no error)"=w352, "Commands in"=w353, "Mirror"=w354) -> ("error out"=w348:errorcluster)  [unwired: 2 in, 2 out]
                            n102 = Add(x=5, y=10) -> (x+y=w349:i32)
                            n103 = Wait (ms)(milliseconds to wait=w349) -> ()  [unwired: 1 out]
                          }
                          frame #3 {
                            # "take offset+initial aberr picture, only one"
                            n104 = local read "EMCCD trigger port"() -> (w357:tag)
                            n105 = call "trig EMCCD.vi"("error in (no error)"=w356, "exp time (ms)"=w358, "lines"=w357) -> ("error out"=w355:errorcluster)
                          }
                          frame #4 {
                            # "other parameters are default in this VI"
                            n106 = Number To Fractional String(number=w374, precision (6)=0) -> (F-format string=w372:string)  [unwired: 2 in]
                            n107 = Concatenate Strings(w376, "_", w372) -> (w361:string)
                            n108 = String To Path(string=w383) -> (path=w385:path)
                            n109 = Concatenate Strings(w383, "\\", w361) -> (w381:string)
                            n110 = String To Path(string=w381) -> (path=w380:path)
                            n111 = call "recon_zern_fileIO_MATLAB.vi"("Number of Phase"="Number of Phase", "Number for average"="Number for average", "Crop Size of image"="Crop Size of image", "Background Value"="Background Value", "Zernike Order"="Zernike Order", "error in (no error)"=w359, "Use GPU"="Use GPU", "Iteration Number"="Iteration Number", "File Name"=w361, "Gamma Value"="Gamma Value", "Path In"=w385, "Show Input"="Show Input", "Path Out"=w380, "Show Recon"="Show Recon") -> ("Zern coef out"=w378:sgl[], "RMSE Value"=w360:dbl, "error out"=w384:errorcluster)  [unwired: 2 in, 1 out]
                            n112 = case shown="False" "Keep Reconstructed Defocus component?" {
                              tunnel: w378 -> [w386 w390]
                              tunnel: [w386 w387] -> w377
                              frame False {
                              }
                              frame True {
                                n113 = Replace Array Subset(array=w390, new element=0.0, index=2) -> (w387:sgl[])
                              }
                            }
                          }
                          frame #5 {
                            w405 = 1
                            # "response time of mirror"
                            n114 = call-poly <vilib>:"Ramp Pattern.vi"("start"=w405, "end"=32, "delta"=w405) -> ("Ramp Pattern"=w403:dbl[])  [unwired: 6 in, 2 out]
                            n115 = call "zern2command_test.vi"("error in (no error)"=w396, "interaction matrix file"=w401, "Zern coef in"=w402, "Zern index in"=w403) -> ("error out"=w395:errorcluster, "Offset positions"=w399:sgl[])  [unwired: 5 in, 1 out]
                            n116 = Add(x=w400, y=w399) -> (x+y=w397:dbl[])
                            n117 = call "PhaseModul apply command.vi"("error in (no error)"=w395, "Commands in"=w397, "Mirror"=w398) -> ("error out"=w391:errorcluster)  [unwired: 2 in, 2 out]
                            n118 = Add(x=5, y=10) -> (x+y=w392:i32)
                            n119 = Wait (ms)(milliseconds to wait=w392) -> ()  [unwired: 1 out]
                          }
                          frame #6 {
                            n120 = for {
                              N: w408 -> [_]
                              tunnel: w409 -> [w412]
                              shift-right: [w410] -> w407
                              shift-left: w406 -> [w411]
                              n121 = local read "EMCCD trigger port"() -> (w413:tag)
                              n122 = call "trig EMCCD.vi"("error in (no error)"=w411, "exp time (ms)"=w412, "lines"=w413) -> ("error out"=w410:errorcluster)
                            }
                            "Error out" <- w407
                          }
                        }
                      }
                    }
                  }
                }
              }
            }
            frame #1 {
              n123 = Concatenate Strings(w415, w414, "_RMSE.txt") -> (w420:string)
              n124 = String To Path(string=w420) -> (path=w419:path)
              n125 = Number To Fractional String(number=w416) -> (F-format string=w417:string[])  [unwired: 3 in]
              n126 = Write to Text File(file (use dialog)=w419, text=w417) -> ()  [unwired: 2 in, 3 out]
            }
          }
        }
      }
    }
    frame #3 {
      n127 = call "Casao dtor.vi"("Casao"=w421) -> ()  [unwired: 6 in, 1 out]
    }
  }
